vi "alert message vua telegram.vi"() -> ()   [LabVIEW 2020]
uses:
  <vilib>/DAQmx/read.llb/DAQmx Read (Digital Bool 1Line 1Point).vi
  <vilib>/DAQmx/create/channels.llb/DAQmx Create Channel (DI-Digital Input).vi
  <vilib>/DAQmx/miscellaneous.llb/DAQmx Fill In Error Info.vi
  <vilib>/ptbypt/NI_PtbyPt.lvlib
  <vilib>/wsapi/NI_WebServices.lvlib
panel:
  in  "lines":tag
  in  "stop":bool
  in  "unescaped string in":string
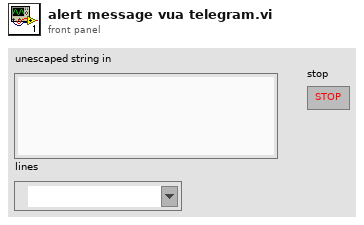
[diagram p1: front panel]
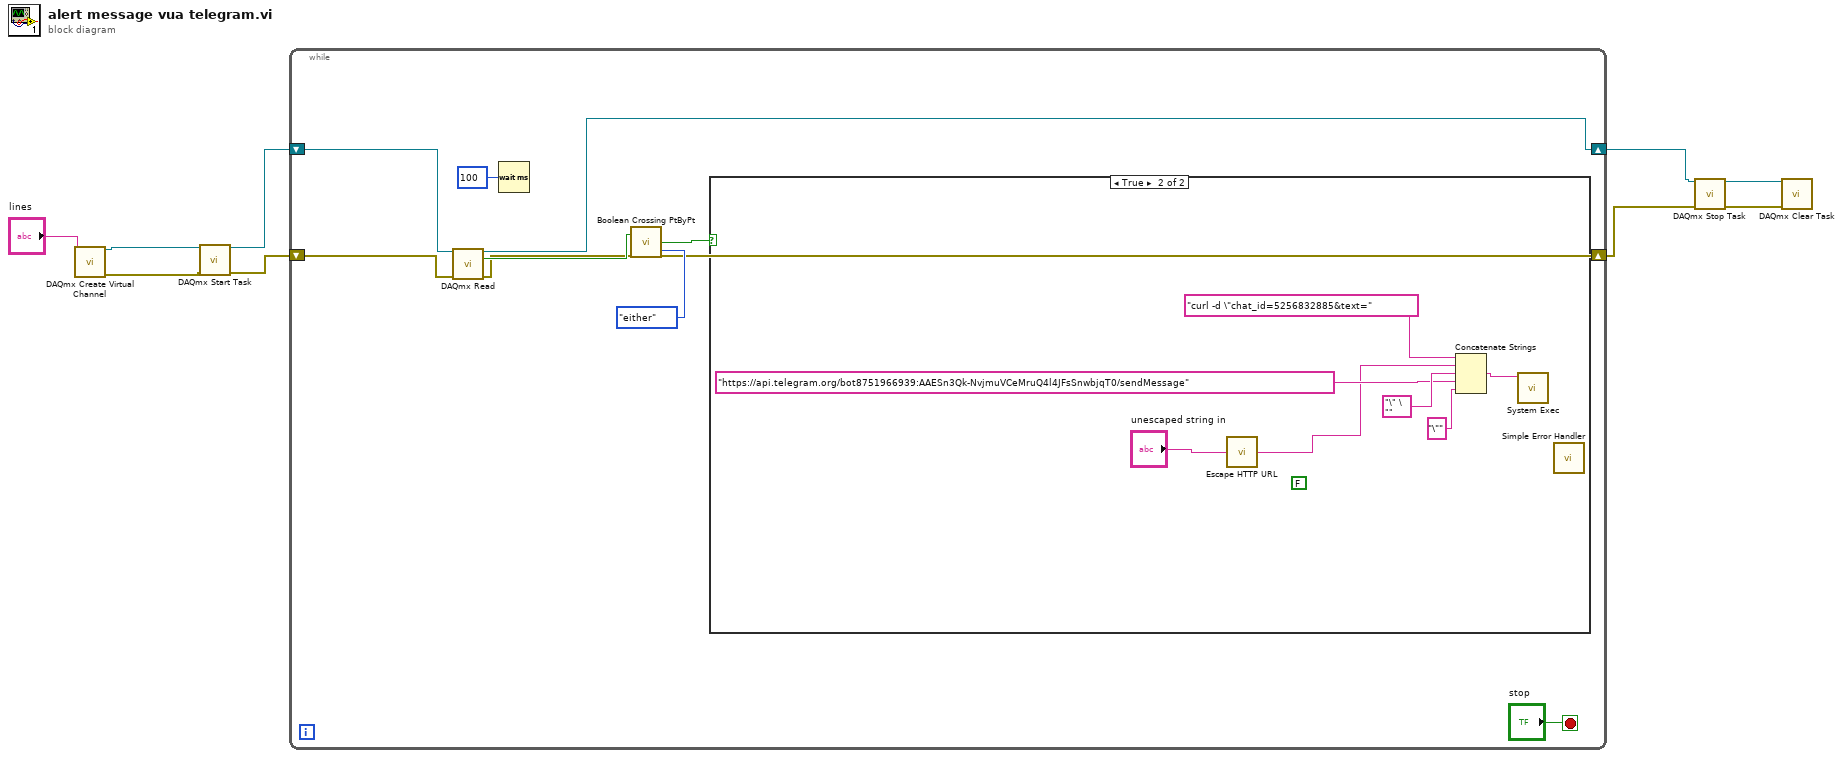
[diagram p0: block diagram]
diagram:
  n1 = call-poly <vilib>:"DAQmx Create Virtual Channel.vi"("lines"="lines") -> ("task out"=w9:refnum<k21>, "error out"=w5:errorcluster)  [unwired: 13 in]
  n2 = call <vilib>:"DAQmx Start Task.vi"("task/channels in"=w9, "error in"=w5) -> ("task out"=w7:refnum<k21>, "error out"=w4:errorcluster)  [unwired: 12 in]
  n3 = while {
    shift-right: [w12] -> w6
    shift-left: w7 -> [w13]
    shift-right: [w10] -> w3
    shift-left: w4 -> [w11]
    stop <- "stop" stop-if-true
    n4 = call-poly <vilib>:"DAQmx Read.vi"("task/channels in"=w13, "error in"=w11) -> ("task out"=w12:refnum<k21>, "data"=w14:bool, "error out"=w10:errorcluster)  [unwired: 11 in]
    n5 = Wait (ms)(milliseconds to wait=u32 100) -> ()  [unwired: 1 out]
    n6 = call <vilib>:"Boolean Crossing PtByPt.vi"("direction"=enum16{"either", "false-true", "true-false"}."either", "input"=w14) -> ("crossing"=w16:bool)  [unwired: 1 in]
    n7 = case shown="True" w16 {
      frame False {
      }
      frame True {
        (unwired) FALSE ("verify server(true)")
        n8 = call <vilib>:"Escape HTTP URL.vi"("unescaped string in"="unescaped string in") -> ("escaped string out"=w20:string)
        n9 = Concatenate Strings("curl -d \"chat_id=5256832885&text=" ("string"), w20, "\" \"" ("string"), "https://api.telegram.org/bot8751966939:AAESn3Qk-NvjmuVCeMruQ4l4JFsSnwbjqT0/sendMessage" ("url"), "\"" ("string")) -> (w19:string)
        n10 = call <vilib>:"System Exec.vi"("command line"=w19) -> ()  [unwired: 7 in, 4 out]
        n11 = call <vilib>:"Simple Error Handler.vi"() -> ()  [unwired: 5 in, 5 out]
      }
    }
  }
  n12 = call <vilib>:"DAQmx Stop Task.vi"("task/channels in"=w6, "error in"=w3) -> ("task out"=w8:refnum<k21>, "error out"=w2:errorcluster)  [unwired: 12 in]
  n13 = call <vilib>:"DAQmx Clear Task.vi"("task in"=w8, "error in"=w2) -> ()  [unwired: 13 in, 1 out]
